vi "MainControlCRIO.vi"() -> ()   [LabVIEW 2017]
uses:
  CRIO_StateEnum.ctl
  CRIO_StateVars.ctl
panel:
  in  "Brake Done":bool
  in  "Coast Done":bool
  in  "Accel Done":bool
  in  "Go Flight":bool
  in  "Setup":bool
  out "State":string
  in  "Port":u16
  in  "Update Rate (ms)":dbl=1.0 min=10.0
  in  "STOP":bool
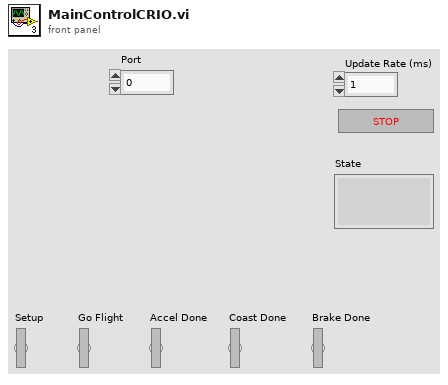
[diagram p1: front panel]
types:
  T1 = typedef "CRIO_StateVars.ctl" = cluster{"connection ID":refnum<k5>, "Connected?":bool, "Transition?":bool}
  T2 = typedef "CRIO_StateEnum.ctl" = enum16{"Init", "Listen", "Wait", "Setup", "Ready to Launch", "Start Flight", "Accelerating", "Coasting", "Braking", "End Flight", "Loading", "Stop"}
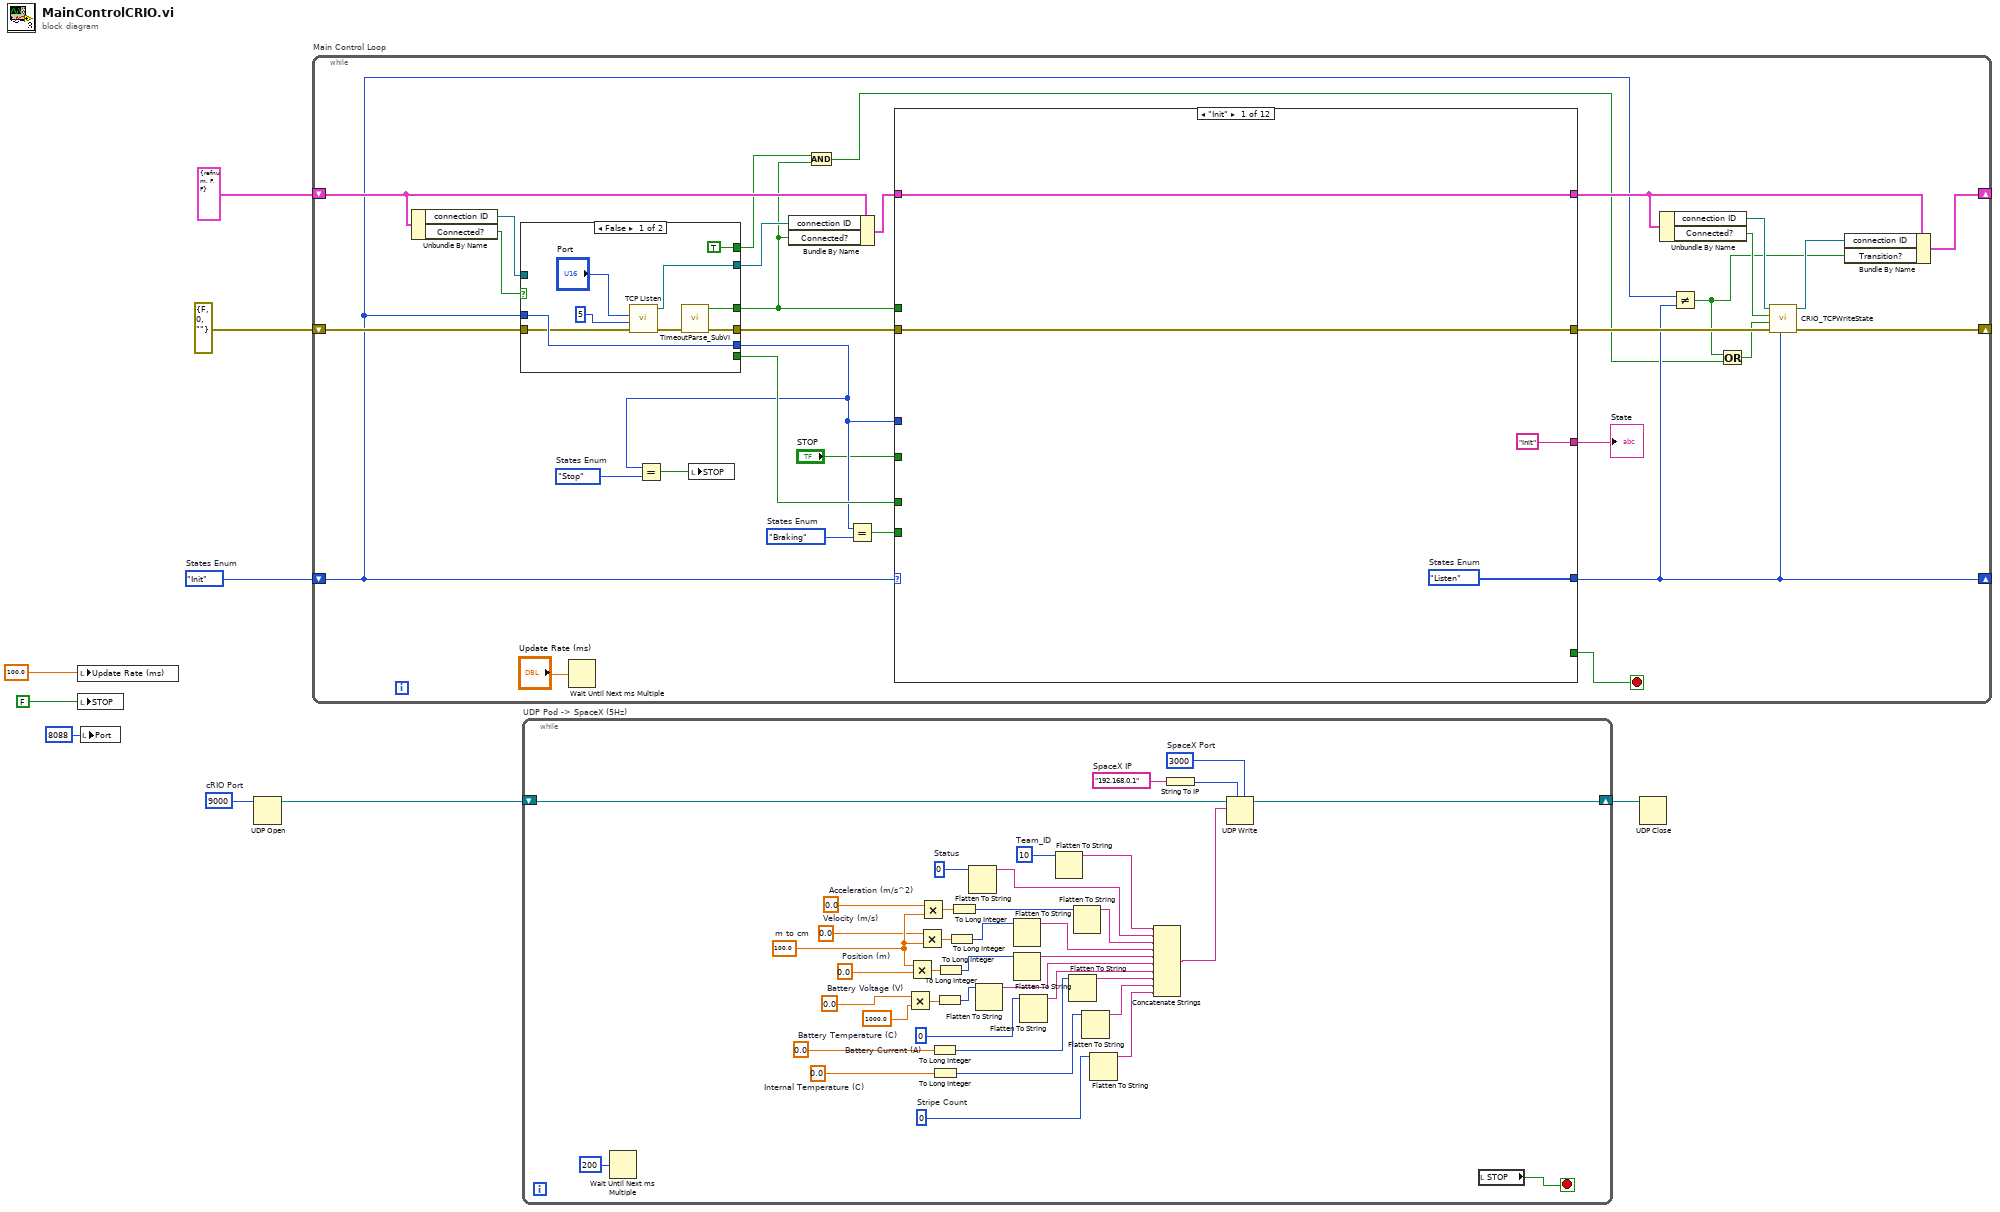
[diagram p0: block diagram]
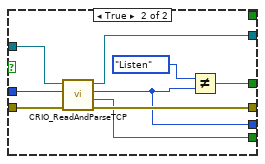
[diagram p2: hidden frame]
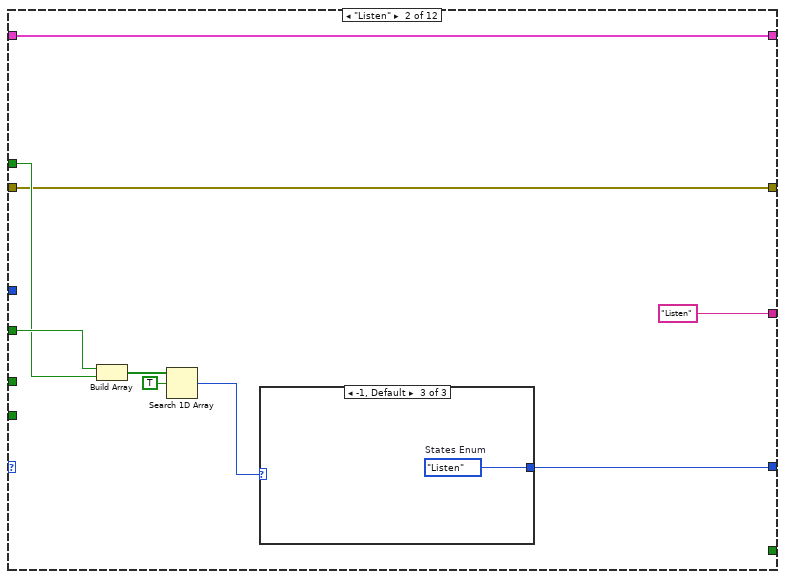
[diagram p3: hidden frame]
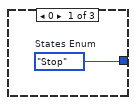
[diagram p4: hidden frame]
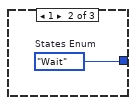
[diagram p5: hidden frame]
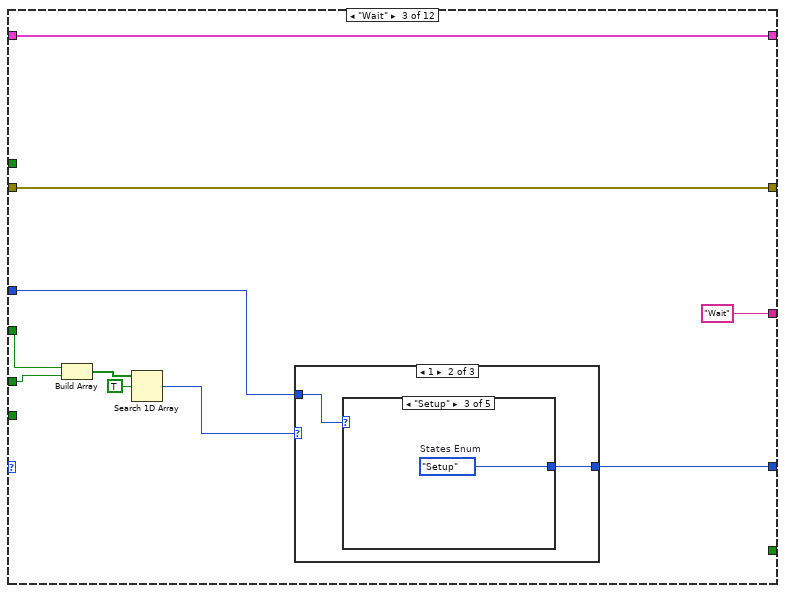
[diagram p6: hidden frame]
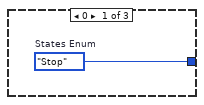
[diagram p7: hidden frame]
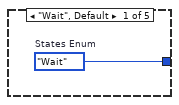
[diagram p8: hidden frame]
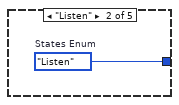
[diagram p9: hidden frame]
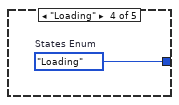
[diagram p10: hidden frame]
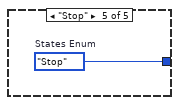
[diagram p11: hidden frame]
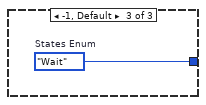
[diagram p12: hidden frame]
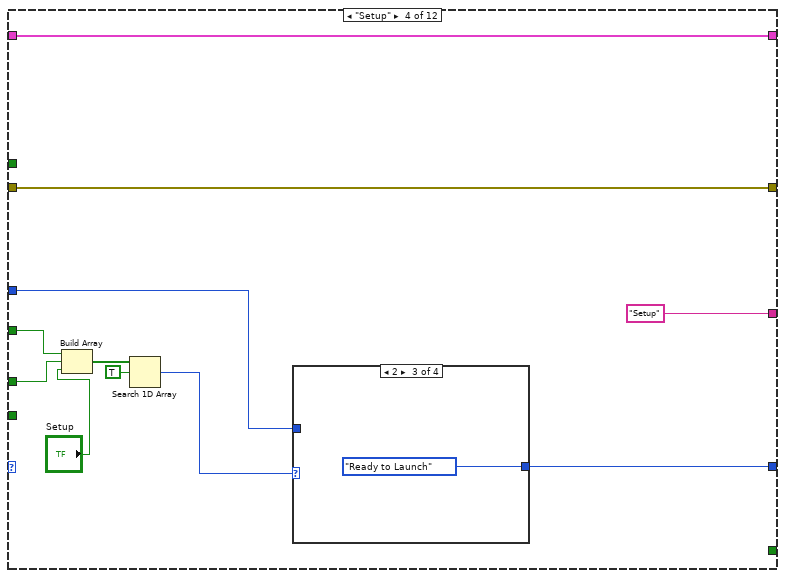
[diagram p13: hidden frame]
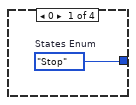
[diagram p14: hidden frame]
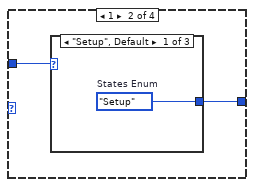
[diagram p15: hidden frame]
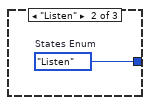
[diagram p16: hidden frame]
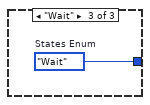
[diagram p17: hidden frame]
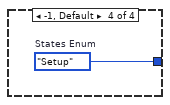
[diagram p18: hidden frame]
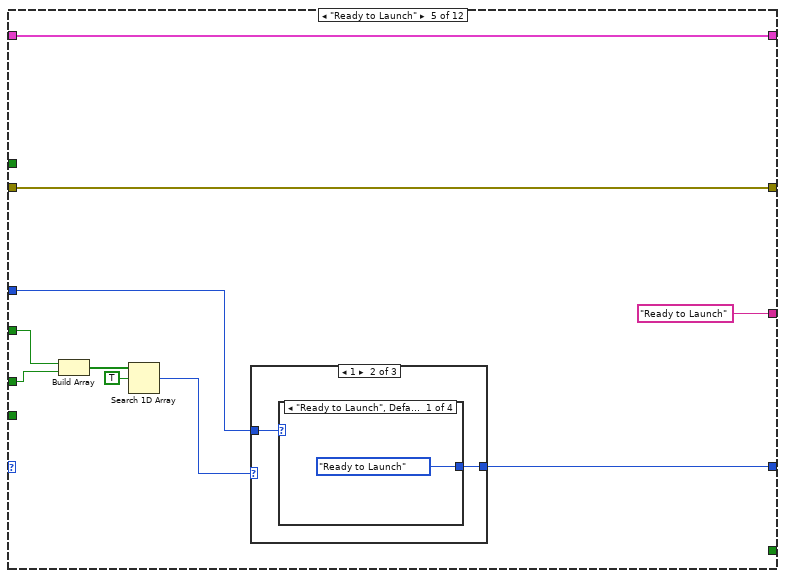
[diagram p19: hidden frame]
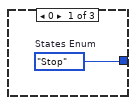
[diagram p20: hidden frame]
diagram:
  w4 = u32 9000  # cRIO Port
  w7 = CRIO_StateEnum."Init"  # States Enum
  n1 = local write "Update Rate (ms)"(100.0) -> ()
  n2 = local write "STOP"(FALSE) -> ()
  n3 = local write "Port"(u16 8088 ("Port")) -> ()
  n4 = UDP Open(11:w4) -> (port=w3:refnum<k16>)  [unwired: 4 in, 2 out]
  n5 = while "Main Control Loop" {
    shift-right: [w15] -> _
    shift-left: w7 -> [w16]
    shift-right: [w18] -> _
    shift-left: T1 {"connection ID"=refnum, "Connected?"=FALSE, "Transition?"=FALSE} -> [w33]
    shift-right: [w22] -> _
    shift-left: errorcluster {"status"=FALSE, "code"=0, "source"=""} ("error constant") -> [w37]
    stop <- w26 stop-if-true
    w28 = CRIO_StateEnum."Stop"  # States Enum
    w30 = CRIO_StateEnum."Braking"  # States Enum
    n6 = Unbundle By Name(w33) -> ("connection ID"=w31:refnum<k5>, "Connected?"=w32:bool)
    n7 = case shown="False" w32 {
      tunnel: [w45 w58] -> w38
      tunnel: w37 -> [w44 w57]
      tunnel: w16 -> [w46 w56]
      tunnel: [w42 w55] -> w35
      tunnel: [w46 w52] -> w27
      tunnel: [_ w54] -> w34
      tunnel: [w43 w53] -> w13
      tunnel: w31 -> [_ w50]
      tunnel: [TRUE _] -> w12
      frame False {
        n8 = call <vilib>:"TCP Listen.vi"("error in (no error)"=w44, "timeout ms (wait forever: -1)"=5, "port"="Port") -> ("error out"=w48:errorcluster, "connection ID"=w42:refnum<k5>)  [unwired: 4 in, 3 out]
        n9 = call "TimeoutParse_SubVI.vi"("error in (no error)"=w48) -> ("error out"=w45:errorcluster, "Connected?"=w43:bool)  [unwired: 9 in]
      }
      frame True {
        n10 = call "CRIO_ReadAndParseTCP.vi"("error in (no error)"=w57, "Curr State"=w56, "TCP Network Connection in"=w50) -> ("error out"=w58:errorcluster, "Update"=w54:bool, "Command State"=w52:T2, "TCP Network Connection out"=w55:refnum<k5>)  [unwired: 5 in]
        n11 = Not Equal?(x=CRIO_StateEnum."Listen" ("Command State"), y=w52) -> (x != y?=w53:bool)
      }
    }
    n12 = Wait Until Next ms Multiple(millisecond multiple="Update Rate (ms)") -> ()  [unwired: 1 out]
    n13 = Equal?(x=w27, y=w28) -> (x = y?=w24:bool)
    n14 = local write "STOP"(w24) -> ()
    n15 = Bundle By Name(cluster=w33, "connection ID"=w35, "Connected?"=w13) -> (w36:T1)
    n16 = And(x=w12, y=w13) -> (x .and. y?=w11:bool)
    n17 = Equal?(x=w27, y=w30) -> (x = y?=w29:bool)
    n18 = case shown="\"Init\"" w16 {
      tunnel: [_ _ _ _ _ _ _ _ _ _ _ TRUE] -> w26
      tunnel: [w61 w68 w81 w101 w119 w136 w148 w167 w186 w202 w223 CRIO_StateEnum."Stop" ("States Enum")] -> w15
      tunnel: w36 -> [w59 w64 w76 w99 w118 w132 w154 w174 w192 w207 w226 w235]
      tunnel: w38 -> [w62 w63 w78 w98 w117 w131 w153 w173 w191 w208 w225 w238]
      tunnel: [w59 w64 w76 w99 w118 w132 w154 w174 w192 w207 w226 w236] -> w19
      tunnel: [w62 w63 w78 w98 w117 w131 w153 w173 w191 w208 w225 w239] -> w23
      tunnel: "STOP" -> [_ w67 w79 w97 w115 w134 w147 w168 w182 w201 w219 _]
      tunnel: ["Init" "Listen" "Wait" "Setup" "Ready to Launch" "Start Flight" "Accelerating" "Coasting" "Braking" "End Flight" "Loading" "Stop"] -> w39
      tunnel: w27 -> [_ _ w75 w95 w113 _ w146 w163 w185 w199 w217 _]
      tunnel: w34 -> [_ _ w77 w96 w114 _ w145 w164 w183 w200 w218 _]
      tunnel: w13 -> [_ w65 _ _ _ _ _ _ _ _ _ _]
      tunnel: w29 -> [_ _ _ _ _ _ w143 w165 _ _ _ _]
      frame "Init" {
        w61 = CRIO_StateEnum."Listen"  # States Enum
      }
      frame "Listen" {
        n19 = Build Array(w67, w65) -> (w71:bool[])
        n20 = Search 1D Array(1D array=w71, element=TRUE) -> (index of element=w69:i32)  [unwired: 1 in]
        n21 = case shown="-1, Default" w69 {
          tunnel: [w72 w73 w74] -> w68
          frame 0 {
            w72 = CRIO_StateEnum."Stop"  # States Enum
          }
          frame 1 {
            w73 = CRIO_StateEnum."Wait"  # States Enum
          }
          frame -1, Default {
            w74 = CRIO_StateEnum."Listen"  # States Enum
          }
        }
      }
      frame "Wait" {
        n22 = Build Array(w79, w77) -> (w84:bool[])
        n23 = Search 1D Array(1D array=w84, element=TRUE) -> (index of element=w82:i32)  [unwired: 1 in]
        n24 = case shown="1" w82 {
          tunnel: [w85 w87 w93] -> w81
          tunnel: w75 -> [_ w86 _]
          frame 0 {
            w85 = CRIO_StateEnum."Stop"  # States Enum
          }
          frame 1 {
            n25 = case shown="\"Setup\"" w86 {
              tunnel: [w88 w89 w90 w91 w92] -> w87
              frame "Wait", Default {
                w88 = CRIO_StateEnum."Wait"  # States Enum
              }
              frame "Listen" {
                w89 = CRIO_StateEnum."Listen"  # States Enum
              }
              frame "Setup" {
                w90 = CRIO_StateEnum."Setup"  # States Enum
              }
              frame "Loading" {
                w91 = CRIO_StateEnum."Loading"  # States Enum
              }
              frame "Stop" {
                w92 = CRIO_StateEnum."Stop"  # States Enum
              }
            }
          }
          frame -1, Default {
            w93 = CRIO_StateEnum."Wait"  # States Enum
          }
        }
      }
      frame "Setup" {
        n26 = Build Array(w97, w96, "Setup") -> (w104:bool[])
        n27 = Search 1D Array(1D array=w104, element=TRUE) -> (index of element=w102:i32)  [unwired: 1 in]
        n28 = case shown="2" w102 {
          tunnel: [w105 w107 CRIO_StateEnum."Ready to Launch" ("States Enum") w112] -> w101
          tunnel: w95 -> [_ w106 _ _]
          frame 0 {
            w105 = CRIO_StateEnum."Stop"  # States Enum
          }
          frame 1 {
            n29 = case shown="\"Setup\", Default" w106 {
              tunnel: [w108 w109 w110] -> w107
              frame "Setup", Default {
                w108 = CRIO_StateEnum."Setup"  # States Enum
              }
              frame "Listen" {
                w109 = CRIO_StateEnum."Listen"  # States Enum
              }
              frame "Wait" {
                w110 = CRIO_StateEnum."Wait"  # States Enum
              }
            }
          }
          frame 2 {
          }
          frame -1, Default {
            w112 = CRIO_StateEnum."Setup"  # States Enum
          }
        }
      }
      frame "Ready to Launch" {
        n30 = Build Array(w115, w114) -> (w122:bool[])
        n31 = Search 1D Array(1D array=w122, element=TRUE) -> (index of element=w120:i32)  [unwired: 1 in]
        n32 = case shown="1" w120 {
          tunnel: [w123 w125 w130] -> w119
          tunnel: w113 -> [_ w124 _]
          frame 0 {
            w123 = CRIO_StateEnum."Stop"  # States Enum
          }
          frame 1 {
            n33 = case shown="\"Ready to Launch\", Default" w124 {
              tunnel: [CRIO_StateEnum."Ready to Launch" ("States Enum") w127 w128 CRIO_StateEnum."Start Flight" ("States Enum")] -> w125
              frame "Ready to Launch", Default {
              }
              frame "Listen" {
                w127 = CRIO_StateEnum."Listen"  # States Enum
              }
              frame "Wait" {
                w128 = CRIO_StateEnum."Wait"  # States Enum
              }
              frame "Start Flight" {
              }
            }
          }
          frame -1, Default {
            w130 = CRIO_StateEnum."Ready to Launch"  # States Enum
          }
        }
      }
      frame "Start Flight" {
        n34 = Build Array(w134, "Go Flight") -> (w139:bool[])
        n35 = Search 1D Array(1D array=w139, element=TRUE) -> (index of element=w137:i32)  [unwired: 1 in]
        n36 = case shown="1" w137 {
          tunnel: [w140 w141 w142] -> w136
          frame 0 {
            w140 = CRIO_StateEnum."Stop"  # States Enum
          }
          frame 1 {
            w141 = CRIO_StateEnum."Accelerating"  # States Enum
          }
          frame -1, Default {
            w142 = CRIO_StateEnum."Start Flight"  # States Enum
          }
        }
      }
      frame "Accelerating" {
        n37 = Build Array(w147, w143, "Accel Done", w145) -> (w151:bool[])
        n38 = Search 1D Array(1D array=w151, element=TRUE) -> (index of element=w149:i32)  [unwired: 1 in]
        n39 = case shown="1" w149 {
          tunnel: [w155 w156 w157 w159 w162] -> w148
          tunnel: w146 -> [_ _ _ w158 _]
          frame 0 {
            w155 = CRIO_StateEnum."Stop"  # States Enum
          }
          frame 1 {
            w156 = CRIO_StateEnum."Braking"  # States Enum
          }
          frame 2 {
            w157 = CRIO_StateEnum."Coasting"  # States Enum
          }
          frame 3 {
            n40 = case shown="\"Accelerating\", Default" w158 {
              tunnel: [CRIO_StateEnum."Accelerating" ("States Enum") w161] -> w159
              frame "Accelerating", Default {
              }
              frame "Braking" {
                w161 = CRIO_StateEnum."Braking"  # States Enum
              }
            }
          }
          frame -1, Default {
            w162 = CRIO_StateEnum."Accelerating"  # States Enum
          }
        }
      }
      frame "Coasting" {
        n41 = Build Array(w168, w165, "Coast Done", w164) -> (w169:bool[])
        n42 = Search 1D Array(1D array=w169, element=TRUE) -> (index of element=w171:i32)  [unwired: 1 in]
        n43 = case shown="0" w171 {
          tunnel: [w175 w176 w178 w181] -> w167
          tunnel: w163 -> [_ _ w177 _]
          frame 0 {
            w175 = CRIO_StateEnum."Stop"  # States Enum
          }
          frame 1, 2 {
            w176 = CRIO_StateEnum."Braking"  # States Enum
          }
          frame 3 {
            n44 = case shown="\"Coasting\", Default" w177 {
              tunnel: [CRIO_StateEnum."Coasting" ("States Enum") w180] -> w178
              frame "Coasting", Default {
              }
              frame "Braking" {
                w180 = CRIO_StateEnum."Braking"  # States Enum
              }
            }
          }
          frame -1, Default {
            w181 = CRIO_StateEnum."Coasting"  # States Enum
          }
        }
      }
      frame "Braking" {
        n45 = Build Array(w182, "Brake Done", w183) -> (w189:bool[])
        n46 = Search 1D Array(1D array=w189, element=TRUE) -> (index of element=w187:i32)  [unwired: 1 in]
        n47 = case shown="2" w187 {
          tunnel: [w193 w194 w196 w198] -> w186
          tunnel: w185 -> [_ _ w195 _]
          frame 0 {
            w193 = CRIO_StateEnum."Stop"  # States Enum
          }
          frame 1 {
            w194 = CRIO_StateEnum."End Flight"  # States Enum
          }
          frame 2 {
            n48 = case shown="\"Braking\", Default" w195 {
              tunnel: [CRIO_StateEnum."Braking" ("States Enum")] -> w196
              frame "Braking", Default {
              }
            }
          }
          frame -1, Default {
            w198 = CRIO_StateEnum."Braking"  # States Enum
          }
        }
      }
      frame "End Flight" {
        n49 = Build Array(w201, w200) -> (w205:bool[])
        n50 = Search 1D Array(1D array=w205, element=TRUE) -> (index of element=w203:i32)  [unwired: 1 in]
        n51 = case shown="1" w203 {
          tunnel: [w209 w211 w216] -> w202
          tunnel: w199 -> [_ w210 _]
          frame 0 {
            w209 = CRIO_StateEnum."Stop"  # States Enum
          }
          frame 1 {
            n52 = case shown="\"End Flight\", Default" w210 {
              tunnel: [CRIO_StateEnum."End Flight" ("States Enum") w213 w214 w215] -> w211
              frame "End Flight", Default {
              }
              frame "Listen" {
                w213 = CRIO_StateEnum."Listen"  # States Enum
              }
              frame "Wait" {
                w214 = CRIO_StateEnum."Wait"  # States Enum
              }
              frame "Loading" {
                w215 = CRIO_StateEnum."Loading"  # States Enum
              }
            }
          }
          frame -1, Default {
            w216 = CRIO_StateEnum."End Flight"  # States Enum
          }
        }
      }
      frame "Loading" {
        n53 = Build Array(w219, w218) -> (w222:bool[])
        n54 = Search 1D Array(1D array=w222, element=TRUE) -> (index of element=w220:i32)  [unwired: 1 in]
        n55 = case shown="1" w220 {
          tunnel: [CRIO_StateEnum."Stop" ("States Enum") w229 CRIO_StateEnum."Loading" ("States Enum")] -> w223
          tunnel: w217 -> [_ w228 _]
          frame 0 {
          }
          frame 1 {
            n56 = case shown="\"Wait\"" w228 {
              tunnel: [CRIO_StateEnum."Loading" ("States Enum") CRIO_StateEnum."Wait" ("States Enum")] -> w229
              frame "Loading", Default {
              }
              frame "Wait" {
              }
            }
          }
          frame -1, Default {
          }
        }
      }
      frame "Stop", Default {
        n57 = Unbundle By Name(w235) -> ("connection ID"=w237:refnum<k5>, "Connected?"=w240:bool)
        n58 = case shown="True" w240 {
          selector: w240 -> [w244 _]
          tunnel: [w246 w250] -> w239
          tunnel: w238 -> [w246 w251]
          tunnel: w237 -> [w245 w249]
          tunnel: [w245 w248] -> w234
          tunnel: [w244 FALSE] -> w233
          frame False {
          }
          frame True {
            n59 = TCP Close Connection(connection ID=w249, error in (no error)=w251) -> (connection ID out=w248:refnum<k5>, error out=w250:errorcluster)  [unwired: 1 in]
          }
        }
        n60 = Bundle By Name(cluster=w235, "connection ID"=w234, "Connected?"=w233) -> (w236:T1)
      }
    }
    "State" <- w39
    n61 = Unbundle By Name(w19) -> ("connection ID"=w21:refnum<k5>, "Connected?"=w17:bool)
    n62 = Not Equal?(x=w16, y=w15) -> (x != y?=w10:bool)
    n63 = Or(x=w10, y=w11) -> (x .or. y?=w14:bool)
    n64 = call "CRIO_TCPWriteState.vi"("Curr State"=w15, "error in (no error)"=w23, "Transition? in"=w14, "Connected?"=w17, "TCP Network Connection in"=w21) -> ("error out"=w22:errorcluster, "TCP Network Connection out"=w20:refnum<k5>)  [unwired: 5 in]
    n65 = Bundle By Name(cluster=w19, "connection ID"=w20, "Transition?"=w10) -> (w18:T1)
  }
  n66 = while "UDP Pod -> SpaceX (5Hz)" {
    shift-right: [w252] -> w2
    shift-left: w3 -> [w253]
    stop <- w262 stop-if-true
    w255 = 0.0  # Internal Temperature (C)
    w259 = 0.0  # Position (m)
    w258 = 0.0  # Velocity (m/s)
    w257 = 0.0  # Battery Voltage (V)
    w256 = 0.0  # Battery Temperature (C)
    w260 = 0.0  # Acceleration (m/s^2)
    w261 = 0  # Status
    w263 = u32 0  # Stripe Count
    w269 = 0  # Battery Current (A)
    w291 = 100.0  # m to cm
    w280 = u8 10  # Team_ID
    w282 = u16 3000  # SpaceX Port
    w285 = "192.168.0.1"  # SpaceX IP
    n67 = Wait Until Next ms Multiple(millisecond multiple=u32 200) -> ()  [unwired: 1 out]
    n68 = Multiply(x=w257, y=1000.0) -> (x*y=w287:dbl)
    n69 = Multiply(x=w291, y=w259) -> (x*y=w288:dbl)
    n70 = Multiply(x=w258, y=w291) -> (x*y=w289:dbl)
    n71 = Multiply(x=w260, y=w291) -> (x*y=w290:dbl)
    n72 = To Long Integer(number=w256) -> (32bit integer=w267:i32)
    n73 = To Long Integer(number=w255) -> (32bit integer=w265:i32)
    n74 = To Long Integer(number=w287) -> (32bit integer=w271:i32)
    n75 = To Long Integer(number=w288) -> (32bit integer=w273:i32)
    n76 = To Long Integer(number=w289) -> (32bit integer=w275:i32)
    n77 = To Long Integer(number=w290) -> (32bit integer=w278:i32)
    n78 = Flatten To String(anything=w261) -> (data string=w279:string)  [unwired: 3 in, 2 out]
    n79 = Flatten To String(anything=w271) -> (data string=w272:string)  [unwired: 3 in, 2 out]
    n80 = Flatten To String(anything=w275) -> (data string=w276:string)  [unwired: 3 in, 2 out]
    n81 = Flatten To String(anything=w273) -> (data string=w274:string)  [unwired: 3 in, 2 out]
    n82 = Flatten To String(anything=w269) -> (data string=w270:string)  [unwired: 3 in, 2 out]
    n83 = Flatten To String(anything=w280) -> (data string=w281:string)  [unwired: 3 in, 2 out]
    n84 = Flatten To String(anything=w267) -> (data string=w268:string)  [unwired: 3 in, 2 out]
    n85 = Flatten To String(anything=w278) -> (data string=w277:string)  [unwired: 3 in, 2 out]
    n86 = Flatten To String(anything=w265) -> (data string=w266:string)  [unwired: 3 in, 2 out]
    n87 = Flatten To String(anything=w263) -> (data string=w264:string)  [unwired: 3 in, 2 out]
    n88 = Concatenate Strings(w281, w279, w277, w276, w274, w272, w270, w268, w266, w264) -> (w284:string)
    n89 = String To IP(1:w285) -> (0:w283:u32)
    n90 = UDP Write(address=w283, port or service name=w282, connection ID=w253, data in=w284) -> (3:w252:refnum<k16>)  [unwired: 2 in, 1 out]
    n91 = local read "STOP"() -> (w262:bool)
  }
  n92 = UDP Close(connection ID=w2) -> ()  [unwired: 1 in, 2 out]
